vi "CentralStorage.Main.vi"   [LabVIEW 2016, in "CentralStorage.lvclass"]
uses:
  CentralStorage.lvclass
  Package Libraries/Message Queue/private/MessageQueue.MessageTypeDef.ctl
  CentralStorage.ReferenceRequest.ctl
  CentralStorage.DataTypes.ctl
  Package ErrorHandling/ErrorHandling.lvclass/ErrorHandling.ctl
  Package ErrorHandling/ErrorHandling.checkForErrorAndHandle.vi
  Package ErrorHandling/ErrorHandling.GetErrorHandler.vi
  <vilib>/Utility/error.llb/Clear Errors.vi
  Package Libraries/StringFunctions/StringFunctions_ReplaceAllBlindSigns.vi
  <vilib>/dlg_ctls.llb/Space Constant.vi
  Package Libraries/TimingFunctions/TimingFunctions_getUtcTimestamp.vi
  <vilib>/Utility/error.llb/Trim Whitespace.vi
  <vilib>/Utility/error.llb/Search and Replace Pattern.vi
  Package ErrorHandling/ErrorHandling.addLastErrorToFile.vi
  Package ErrorHandling/ErrorHandling.lvclass
types:
  T1 = typedef "MessageQueue.MessageTypeDef.ctl" = cluster{"Message":string, "Data":variant}
  T2 = typedef "CentralStorage.lvclass/CentralStorage.ReferenceRequest.ctl" = cluster{"Caller":string, "DataType":T3, "Data":variant}
  T3 = typedef "CentralStorage.lvclass/CentralStorage.DataTypes.ctl" = enum16{"Variant Array", "Variant", "Waveform"}
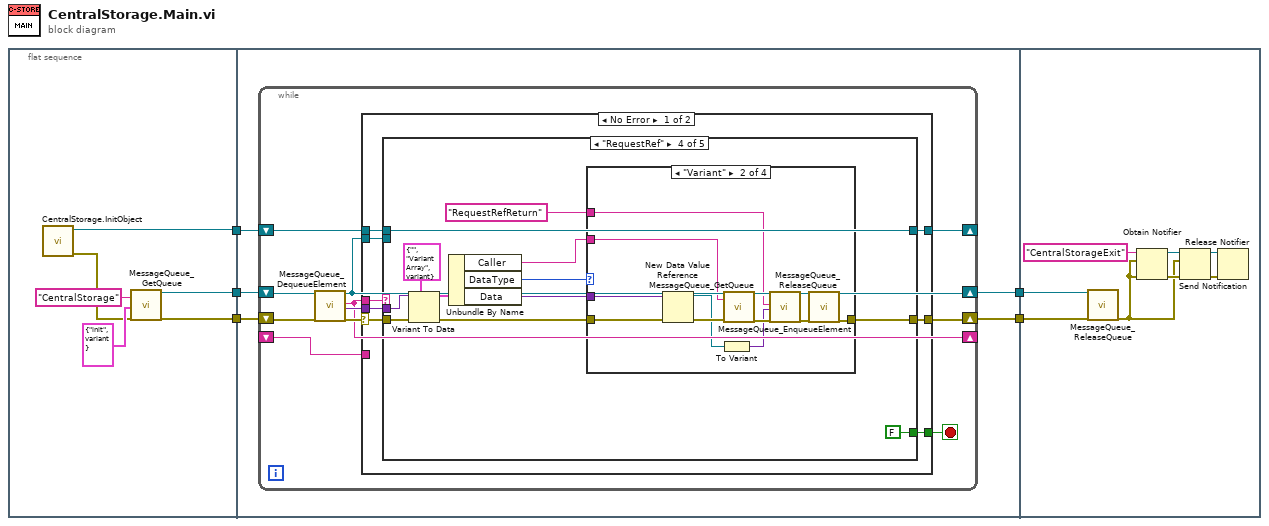
[diagram p0: block diagram]
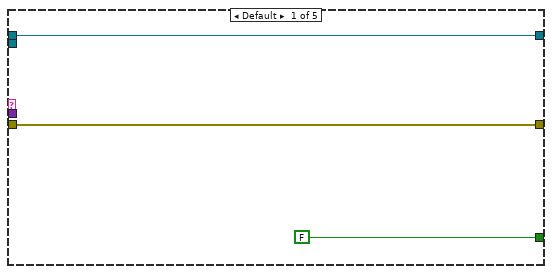
[diagram p2: hidden frame]
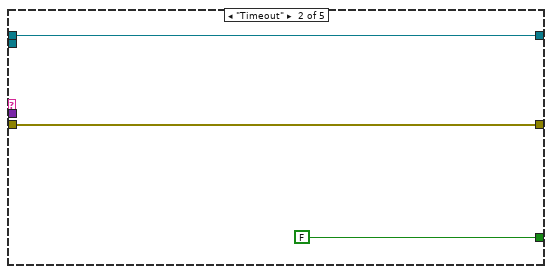
[diagram p3: hidden frame]
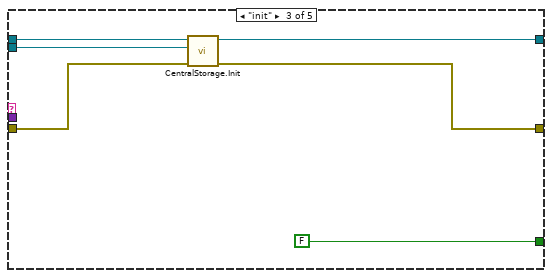
[diagram p4: hidden frame]
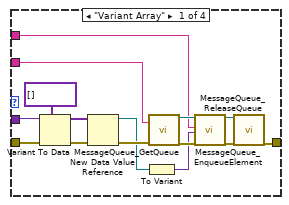
[diagram p5: hidden frame]
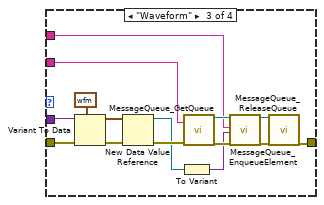
[diagram p6: hidden frame]
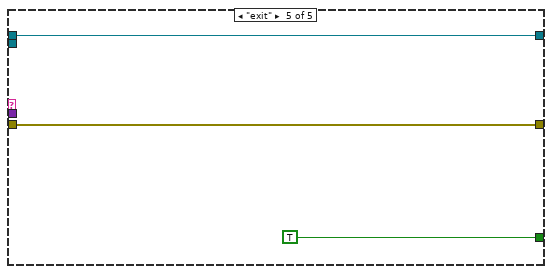
[diagram p8: hidden frame]
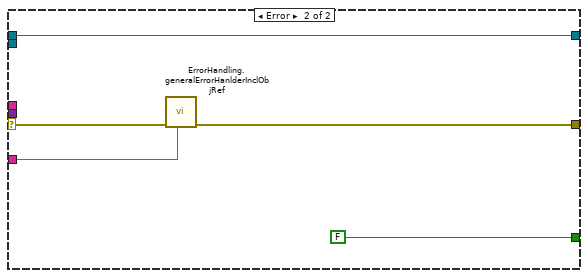
[diagram p9: hidden frame]
diagram:
  n1 = flat-sequence {
    tunnel: [w6] -> w5
    tunnel: [w10] -> w4
    tunnel: [w9] -> w3
    tunnel: w5 -> [w14]
    tunnel: w4 -> [w16]
    tunnel: w3 -> [w15]
    tunnel: [w13] -> w2
    tunnel: [w12] -> w1
    tunnel: w2 -> [w118]
    tunnel: w1 -> [w117]
    frame #0 {
      n2 = call "CentralStorage.InitObject.vi"() -> ("Error out"=w7:errorcluster, "CentralStorage"=w6:refnum<data-value>)  [unwired: 10 in]
      n3 = call "MessageQueue_GetQueue.vi"("Name"="CentralStorage", "OptionalInitValue"=T1 {"Message"="init", "Data"=variant}, "ErrorIn"=w7) -> ("QueueOut"=w10:refnum<queue>, "ErrorOut"=w9:errorcluster)  [unwired: 14 in, 1 out]
    }
    frame #1 {
      n4 = while {
        shift-right: [w22] -> _
        shift-left: w14 -> [w23]
        shift-right: [w20] -> w13
        shift-left: w15 -> [w27]
        shift-right: [w17] -> w12
        shift-left: w16 -> [w26]
        shift-right: [w19] -> _
        shift-left: _ -> [w18]
        stop <- w21 stop-if-true
        n5 = call "MessageQueue_DequeueElement.vi"("QueueIn"=w26, "ErrorIn"=w27) -> ("QueueOut"=w17:refnum<queue>, "Message"=w19:string, "Data"=w24:variant, "ErrorOut"=w25:errorcluster)  [unwired: 13 in, 1 out]
        n6 = case shown="No Error" w25 {
          selector: w25 -> [w33 w108]
          tunnel: w19 -> [w35 _]
          tunnel: w24 -> [w34 _]
          tunnel: w23 -> [w32 w110]
          tunnel: [w31 w110] -> w22
          tunnel: [w30 w107] -> w20
          tunnel: [w29 FALSE] -> w21
          tunnel: w18 -> [_ w106]
          tunnel: w17 -> [w28 _]
          frame No Error {
            n7 = case shown="\"RequestRef\"" w35 {
              tunnel: w34 -> [_ _ _ w59 _]
              tunnel: w33 -> [w37 w39 w46 w58 w103]
              tunnel: w32 -> [w38 w40 w43 w56 w104]
              tunnel: [w38 w40 w44 w56 w104] -> w31
              tunnel: [w37 w39 w45 w51 w103] -> w30
              tunnel: [FALSE FALSE FALSE FALSE TRUE] -> w29
              tunnel: w28 -> [_ _ w42 _ _]
              frame Default {
              }
              frame "Timeout" {
              }
              frame "init" {
                n8 = call "CentralStorage.Init.vi"("error in (no error)"=w46, "OwnQueue"=w42, "CentralStorage in"=w43) -> ("error out"=w45:errorcluster, "CentralStorage out"=w44:refnum<data-value>)  [unwired: 7 in]
              }
              frame "RequestRef" {
                n9 = Variant To Data(error in=w58, type=T2 {"Caller"="", "DataType"=enum."Variant Array", "Data"=variant} ("output cluster"), Variant=w59) -> (data=w54:T2, error out=w52:errorcluster)
                n10 = Unbundle By Name(w54) -> ("Caller"=w49:string, "DataType"=w53:T3, "Data"=w50:variant)
                n11 = case shown="\"Variant\"" w53 {
                  tunnel: w52 -> [w72 w75 w100 w102]
                  tunnel: [w67 w84 w95 w102] -> w51
                  tunnel: w50 -> [w74 w76 w101 _]
                  tunnel: w49 -> [w64 w81 w92 _]
                  tunnel: "RequestRefReturn" ("Caller") -> [w60 w77 w88 _]
                  frame "Variant Array" {
                    n12 = Variant To Data(error in=w72, type=variant[] [], Variant=w74) -> (data=w70:variant[], error out=w71:errorcluster)
                    n13 = New Data Value Reference(data value=w70, error in=w71) -> (data value reference=w62:refnum<data-value>, error out=w69:errorcluster)
                    n14 = To Variant(anything=w62) -> (Variant=w61:variant)
                    n15 = call "MessageQueue_GetQueue.vi"("Name"=w64, "ErrorIn"=w69) -> ("QueueOut"=w63:refnum<queue>, "ErrorOut"=w65:errorcluster)  [unwired: 15 in, 1 out]
                    n16 = call "MessageQueue_EnqueueElement.vi"("QueueIn"=w63, "Message"=w60, "Data"=w61, "ErrorIn"=w65) -> ("QueueOut"=w68:refnum<queue>, "ErrorOut"=w66:errorcluster)  [unwired: 14 in]
                    n17 = call "MessageQueue_ReleaseQueue.vi"("QueueIn"=w68, "ErrorIn"=w66) -> ("ErrorOut"=w67:errorcluster)  [unwired: 15 in, 2 out]
                  }
                  frame "Variant" {
                    n18 = New Data Value Reference(data value=w76, error in=w75) -> (data value reference=w79:refnum<data-value>, error out=w86:errorcluster)
                    n19 = To Variant(anything=w79) -> (Variant=w78:variant)
                    n20 = call "MessageQueue_GetQueue.vi"("Name"=w81, "ErrorIn"=w86) -> ("QueueOut"=w80:refnum<queue>, "ErrorOut"=w82:errorcluster)  [unwired: 15 in, 1 out]
                    n21 = call "MessageQueue_EnqueueElement.vi"("QueueIn"=w80, "Message"=w77, "Data"=w78, "ErrorIn"=w82) -> ("QueueOut"=w85:refnum<queue>, "ErrorOut"=w83:errorcluster)  [unwired: 14 in]
                    n22 = call "MessageQueue_ReleaseQueue.vi"("QueueIn"=w85, "ErrorIn"=w83) -> ("ErrorOut"=w84:errorcluster)  [unwired: 15 in, 2 out]
                  }
                  frame "Waveform" {
                    n23 = Variant To Data(error in=w100, type=waveform(dbl) {"t0"=timestamp(0 s since 1904-01-01), "dt"=1.0, "Y"=[]} ("waveform"), Variant=w101) -> (data=w98:waveform(dbl), error out=w99:errorcluster)
                    n24 = New Data Value Reference(data value=w98, error in=w99) -> (data value reference=w90:refnum<data-value>, error out=w97:errorcluster)
                    n25 = To Variant(anything=w90) -> (Variant=w89:variant)
                    n26 = call "MessageQueue_GetQueue.vi"("Name"=w92, "ErrorIn"=w97) -> ("QueueOut"=w91:refnum<queue>, "ErrorOut"=w93:errorcluster)  [unwired: 15 in, 1 out]
                    n27 = call "MessageQueue_EnqueueElement.vi"("QueueIn"=w91, "Message"=w88, "Data"=w89, "ErrorIn"=w93) -> ("QueueOut"=w96:refnum<queue>, "ErrorOut"=w94:errorcluster)  [unwired: 14 in]
                    n28 = call "MessageQueue_ReleaseQueue.vi"("QueueIn"=w96, "ErrorIn"=w94) -> ("ErrorOut"=w95:errorcluster)  [unwired: 15 in, 2 out]
                  }
                  frame Default {
                  }
                }
              }
              frame "exit" {
              }
            }
          }
          frame Error {
            n29 = call "ErrorHandling.generalErrorHanlderInclObjRef.vi"("LastCommand(optional)"=w106, "error in"=w108) -> ("error out"=w107:errorcluster)  [unwired: 7 in, 2 out]
          }
        }
      }
    }
    frame #2 {
      n30 = call "MessageQueue_ReleaseQueue.vi"("QueueIn"=w117, "ErrorIn"=w118) -> ("ErrorOut"=w113:errorcluster)  [unwired: 15 in, 2 out]
      n31 = Obtain Notifier(name (unnamed)="CentralStorageExit", notification data type=w113, error in (no error)=w113) -> (notifier out=w114:refnum<notifier>, error out=w115:errorcluster)  [unwired: 1 in, 1 out]
      n32 = Send Notification(notification=w113, notifier=w114, error in (no error)=w115) -> (notifier out=w111:refnum<notifier>, error out=w112:errorcluster)
      n33 = Release Notifier(notifier=w111, error in (no error)=w112) -> ()  [unwired: 1 in, 3 out]
    }
  }
